vi "Check Relay State.vi"(8 "error in (no error)":errorcluster, 10 "relay string":string, 11 "Route Manager in":refnum<class "Route Manager.lvclass">) -> (0 "error out":errorcluster, 2 "position":T1=10 items=["Open"=10, "Closed"=11])   [LabVIEW 2015, in "Route Manager.lvclass"]
uses:
  Route Manager.lvclass
  Position.ctl
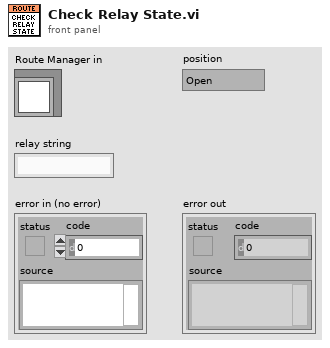
[diagram p1: front panel]
types:
  T1 = typedef "Route Manager.lvclass/Position.ctl" = i32
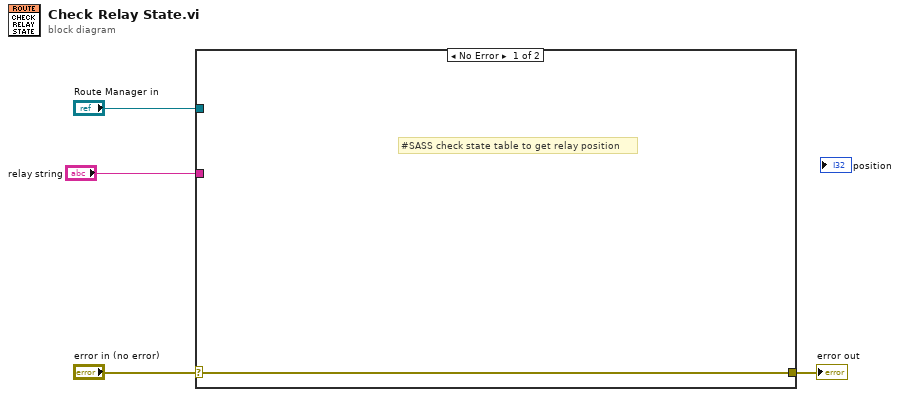
[diagram p0: block diagram]
diagram:
  n1 = case shown="No Error" "error in (no error)" {
    selector: "error in (no error)" -> [w5 w6]
    tunnel: [w5 w6] -> w3
    tunnel: "Route Manager in" -> [_ _]
    tunnel: "relay string" -> [_ _]
    frame No Error {
      # "#SASS check state table to get relay position"
    }
    frame Error {
    }
  }
  "error out" <- w3
